vi "DMARS_Frame_v2_write.vi"(11 "DMARS":dbl[](array[numeric])) -> (0 "No DMARS string":bool, 3 "string_Out":string)   [LabVIEW 2017]
panel:
  out "SubFrame":u8
  out "milisec":u16 format="%x"
  out "sec":u16 format="%x"
  out "size(s)":i32
  out "output array":u8[](array[numeric]) format="%x"
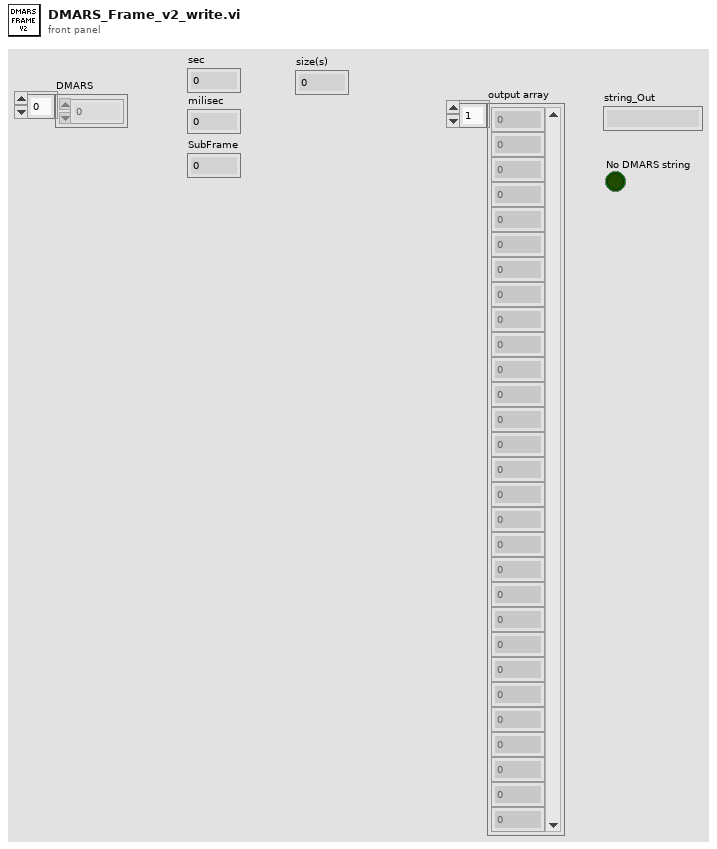
[diagram p1: front panel]
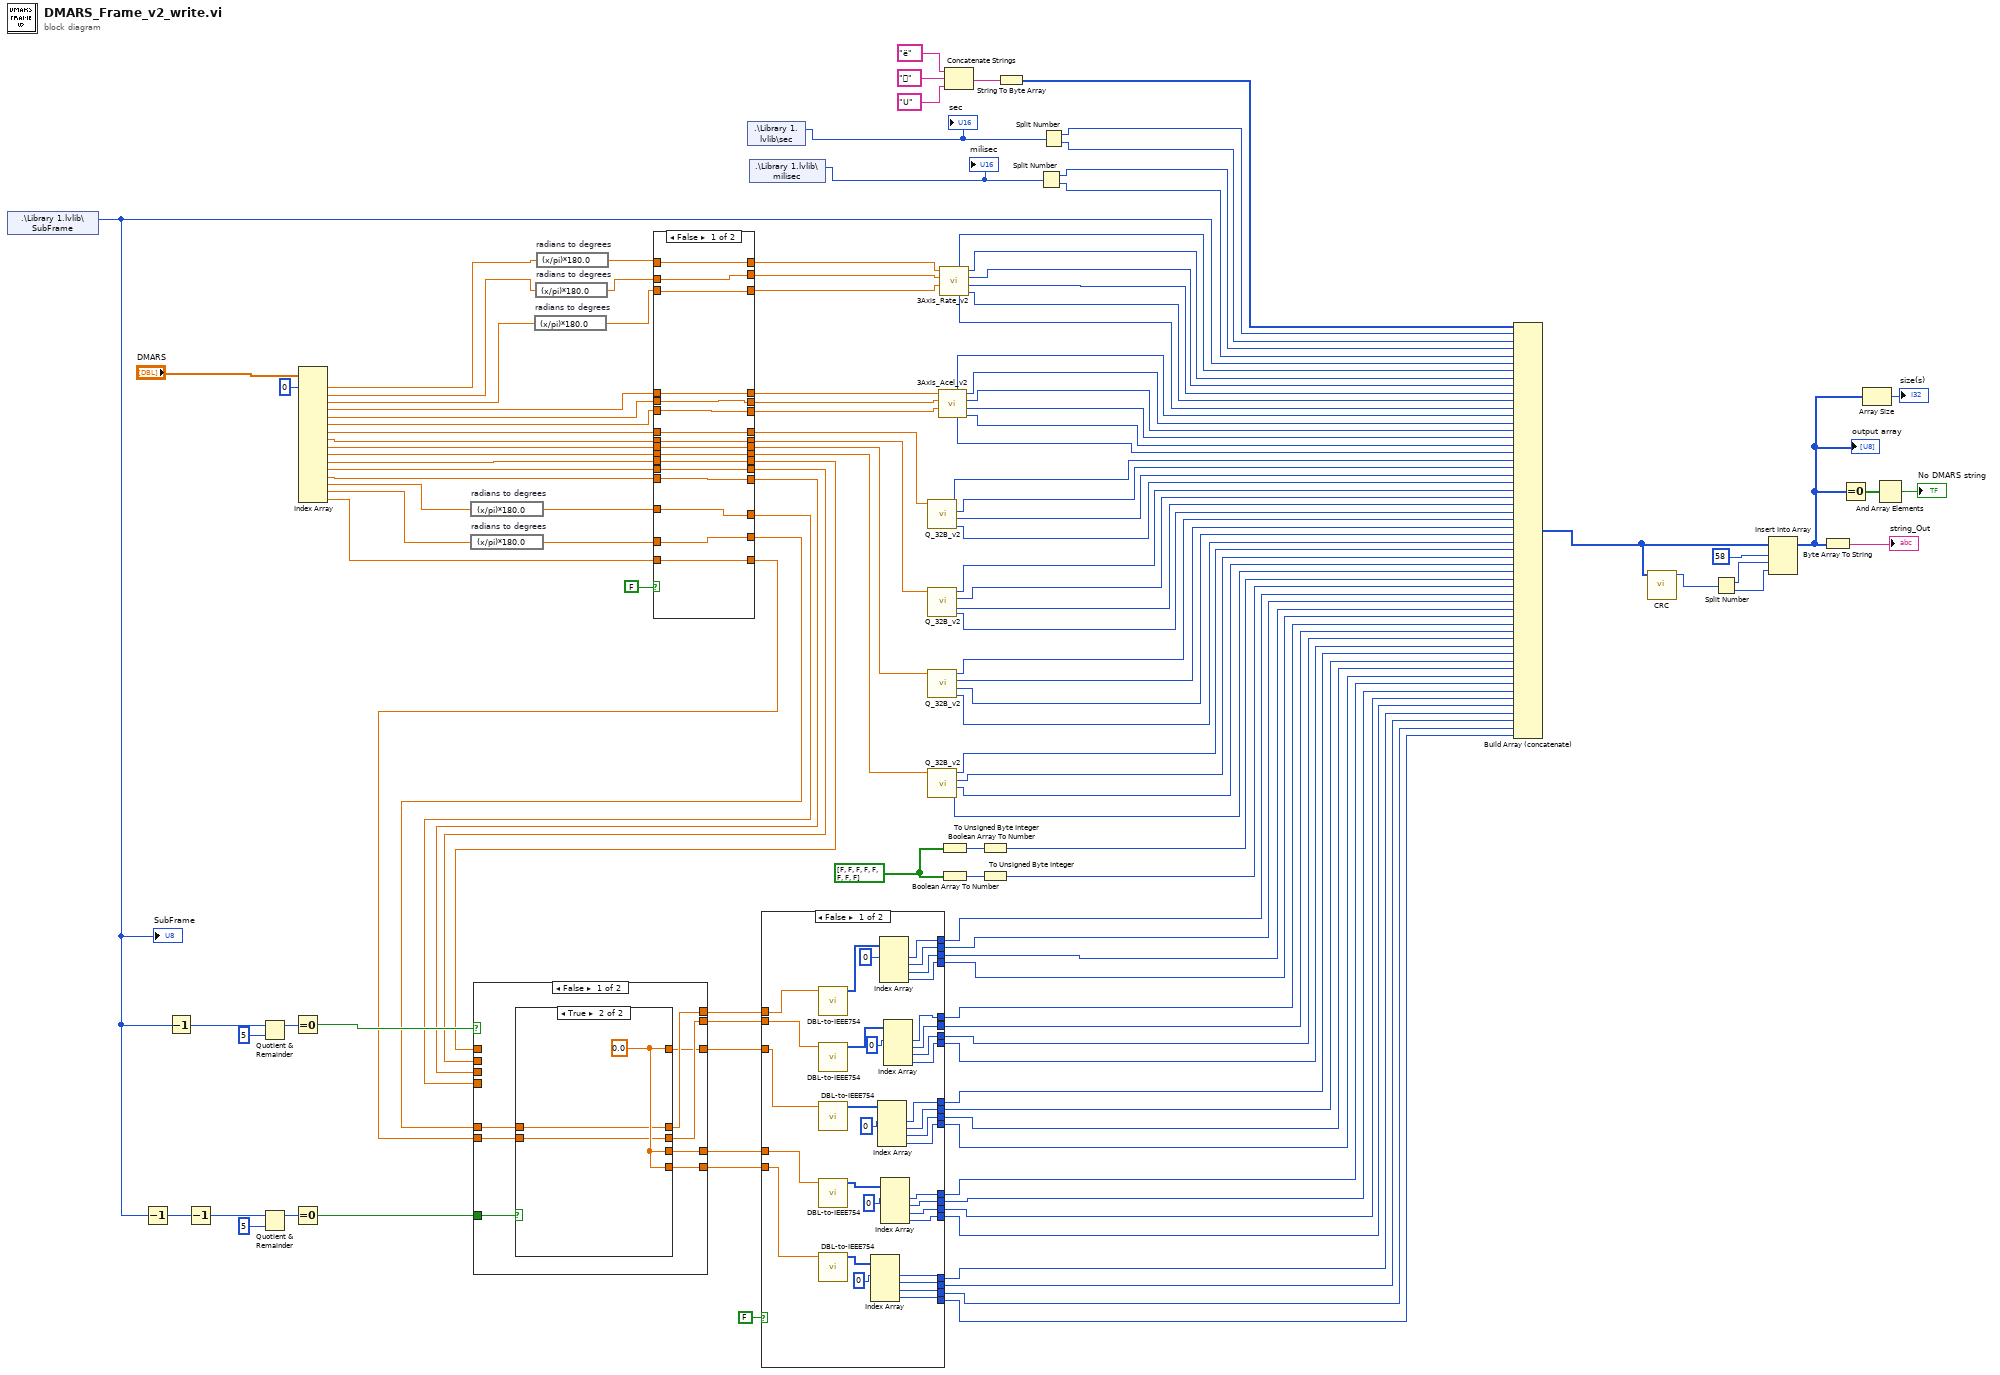
[diagram p0: block diagram]
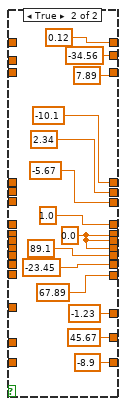
[diagram p2: hidden frame]
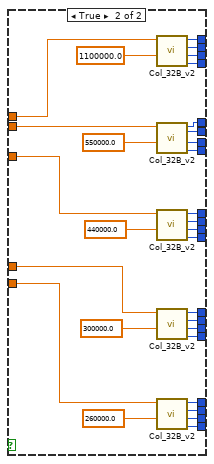
[diagram p3: hidden frame]
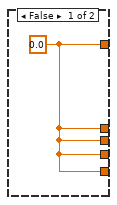
[diagram p4: hidden frame]
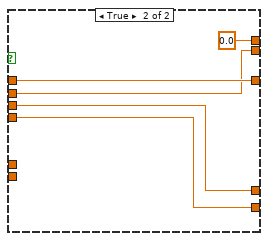
[diagram p5: hidden frame]
diagram:
  w64 = bool[] [FALSE, FALSE, FALSE, FALSE, FALSE, FALSE, FALSE, FALSE] ("Byte 36")
  n1 = shared-variable ".\\Library 1.lvlib\\SubFrame"() -> (w52:u8)  [unwired: 1 in, 1 out]
  "SubFrame" <- w52
  n2 = Decrement(x=w52) -> (x-1=w53:u8)
  n3 = Decrement(x=w52) -> (x-1=w57:u8)
  n4 = Decrement(x=w53) -> (x-1=w56:u8)
  n5 = Quotient & Remainder(x=w57, y=u8 5) -> (x-y*floor(x/y)=w59:u8)  [unwired: 1 out]
  n6 = Quotient & Remainder(x=w56, y=u8 5) -> (x-y*floor(x/y)=w55:u8)  [unwired: 1 out]
  n7 = Equal To 0?(x=w59) -> (x = 0?=w58:bool)
  n8 = Equal To 0?(x=w55) -> (x = 0?=w46:bool)
  n9 = Index Array(array="DMARS", index #1=0 ("index")) -> (element #1=w11:dbl, element #2=w9:dbl, element #3=w8:dbl, element #4=w37:dbl, element #5=w35:dbl, element #6=w33:dbl, element #7=w31:dbl, element #8=w29:dbl, element #9=w28:dbl, element #10=w25:dbl, element #11=w23:dbl, element #12=w21:dbl, element #13=w19:dbl, element #14=w45:dbl, element #15=w44:dbl, element #16=w13:dbl)  [unwired: 15 in]
  n10 = expression code="(x/pi)*180.0" "radians to degrees"(w45) -> (w17:dbl)
  n11 = expression code="(x/pi)*180.0" "radians to degrees"(w44) -> (w15:dbl)
  n12 = expression code="(x/pi)*180.0" "radians to degrees"(w8) -> (w6:dbl)
  n13 = expression code="(x/pi)*180.0" "radians to degrees"(w9) -> (w7:dbl)
  n14 = expression code="(x/pi)*180.0" "radians to degrees"(w11) -> (w10:dbl)
  n15 = case shown="False" FALSE {
    tunnel: [w146 0.12 ("Numeric")] -> w41
    tunnel: w10 -> [w146 _]
    tunnel: [w145 -34.56 ("Numeric")] -> w40
    tunnel: w7 -> [w145 _]
    tunnel: [w131 7.89 ("Numeric")] -> w39
    tunnel: w6 -> [w131 _]
    tunnel: [w144 -10.1 ("Numeric")] -> w38
    tunnel: w37 -> [w144 _]
    tunnel: [w143 2.34 ("Numeric")] -> w36
    tunnel: w35 -> [w143 _]
    tunnel: [w142 -5.67 ("Numeric")] -> w34
    tunnel: w33 -> [w142 _]
    tunnel: [w141 1.0 ("Numeric")] -> w32
    tunnel: w31 -> [w141 _]
    tunnel: [w140 w153] -> w30
    tunnel: w29 -> [w140 _]
    tunnel: w28 -> [w139 _]
    tunnel: [w139 w153] -> w27
    tunnel: [w138 w153] -> w26
    tunnel: w25 -> [w138 _]
    tunnel: [w137 89.1 ("Numeric")] -> w24
    tunnel: w23 -> [w137 _]
    tunnel: [w136 -23.45 ("Numeric")] -> w22
    tunnel: w21 -> [w136 _]
    tunnel: [w135 67.89 ("Numeric")] -> w20
    tunnel: w19 -> [w135 _]
    tunnel: [w134 -1.23 ("Numeric")] -> w18
    tunnel: w17 -> [w134 _]
    tunnel: [w133 45.67 ("Numeric")] -> w16
    tunnel: w15 -> [w133 _]
    tunnel: [w132 -8.9 ("Numeric")] -> w14
    tunnel: w13 -> [w132 _]
    frame False {
    }
    frame True {
      w153 = 0.0 ("Numeric")
    }
  }
  n16 = case shown="False" w58 {
    tunnel: w24 -> [_ w176]
    tunnel: w22 -> [_ w175]
    tunnel: w20 -> [_ w174]
    tunnel: w18 -> [_ w173]
    tunnel: [w165 0.0] -> w51
    tunnel: [w163 w176] -> w50
    tunnel: [w164 w175] -> w49
    tunnel: [w162 w174] -> w48
    tunnel: [w161 w173] -> w47
    tunnel: w46 -> [w168 _]
    tunnel: w16 -> [w167 _]
    tunnel: w14 -> [w166 _]
    frame False {
      n17 = case shown="True" w168 {
        tunnel: w167 -> [_ w171]
        tunnel: w166 -> [_ w170]
        tunnel: [w169 w171] -> w165
        tunnel: [w169 w170] -> w164
        tunnel: [w169 w172] -> w163
        tunnel: [w169 w172] -> w162
        tunnel: [w169 w172] -> w161
        frame False {
          w169 = 0.0
        }
        frame True {
          w172 = 0.0
        }
      }
    }
    frame True {
    }
  }
  n18 = shared-variable ".\\Library 1.lvlib\\sec"() -> (w63:u16)  [unwired: 1 in, 1 out]
  "sec" <- w63
  n19 = shared-variable ".\\Library 1.lvlib\\milisec"() -> (w62:u16)  [unwired: 1 in, 1 out]
  "milisec" <- w62
  n20 = case shown="False" FALSE {
    tunnel: [w181 w242] -> w125
    tunnel: [w178 w241] -> w124
    tunnel: [w179 w240] -> w123
    tunnel: [w180 w239] -> w122
    tunnel: [w182 w238] -> w121
    tunnel: [w183 w237] -> w120
    tunnel: [w184 w236] -> w119
    tunnel: [w185 w235] -> w118
    tunnel: [w190 w234] -> w117
    tunnel: [w191 w233] -> w116
    tunnel: [w192 w232] -> w115
    tunnel: [w193 w231] -> w114
    tunnel: [w196 w230] -> w113
    tunnel: [w197 w229] -> w112
    tunnel: [w198 w228] -> w111
    tunnel: [w199 w227] -> w110
    tunnel: [w203 w226] -> w109
    tunnel: [w204 w225] -> w108
    tunnel: [w205 w224] -> w107
    tunnel: [w206 w223] -> w106
    tunnel: w51 -> [w212 w222]
    tunnel: w50 -> [w210 w221]
    tunnel: w49 -> [w211 w220]
    tunnel: w48 -> [w209 w219]
    tunnel: w47 -> [w208 w218]
    frame False {
      n21 = call "DBL-to-IEEE754.vi"("Input_DBL"=w212) -> ("Output_U8"=w207:u8[])  [unwired: 10 in]
      n22 = call "DBL-to-IEEE754.vi"("Input_DBL"=w211) -> ("Output_U8"=w201:u8[])  [unwired: 10 in]
      n23 = call "DBL-to-IEEE754.vi"("Input_DBL"=w210) -> ("Output_U8"=w194:u8[])  [unwired: 10 in]
      n24 = call "DBL-to-IEEE754.vi"("Input_DBL"=w209) -> ("Output_U8"=w186:u8[])  [unwired: 10 in]
      n25 = call "DBL-to-IEEE754.vi"("Input_DBL"=w208) -> ("Output_U8"=w187:u8[])  [unwired: 10 in]
      n26 = Index Array(array=w187, index #1=0 ("index")) -> (element #1=w181:u8, element #2=w180:u8, element #3=w179:u8, element #4=w178:u8)  [unwired: 3 in]
      n27 = Index Array(array=w194, index #1=0 ("index")) -> (element #1=w193:u8, element #2=w192:u8, element #3=w191:u8, element #4=w190:u8)  [unwired: 3 in]
      n28 = Index Array(array=w207, index #1=0 ("index")) -> (element #1=w206:u8, element #2=w205:u8, element #3=w204:u8, element #4=w203:u8)  [unwired: 3 in]
      n29 = Index Array(array=w186, index #1=0 ("index")) -> (element #1=w185:u8, element #2=w184:u8, element #3=w183:u8, element #4=w182:u8)  [unwired: 3 in]
      n30 = Index Array(array=w201, index #1=0 ("index")) -> (element #1=w199:u8, element #2=w198:u8, element #3=w197:u8, element #4=w196:u8)  [unwired: 3 in]
    }
    frame True {
      n31 = call "Col_32B_v2.vi"("Ref"=1100000.0, "Col"=w222) -> ("LL"=w226:u8, "LH"=w225:u8, "HL"=w224:u8, "HH"=w223:u8)  [unwired: 6 in]
      n32 = call "Col_32B_v2.vi"("Ref"=550000.0, "Col"=w220) -> ("LL"=w230:u8, "LH"=w229:u8, "HL"=w228:u8, "HH"=w227:u8)  [unwired: 6 in]
      n33 = call "Col_32B_v2.vi"("Ref"=440000.0, "Col"=w221) -> ("LL"=w234:u8, "LH"=w233:u8, "HL"=w232:u8, "HH"=w231:u8)  [unwired: 6 in]
      n34 = call "Col_32B_v2.vi"("Ref"=300000.0, "Col"=w219) -> ("LL"=w238:u8, "LH"=w237:u8, "HL"=w236:u8, "HH"=w235:u8)  [unwired: 6 in]
      n35 = call "Col_32B_v2.vi"("Ref"=260000.0, "Col"=w218) -> ("LL"=w241:u8, "LH"=w240:u8, "HL"=w239:u8, "HH"=w242:u8)  [unwired: 6 in]
    }
  }
  n36 = call "Q_32B_v2.vi"("Q_32B"=w32) -> ("LL"=w91:u8, "HL"=w90:u8, "LH"=w89:u8, "HH"=w88:u8)  [unwired: 7 in]
  n37 = call "Q_32B_v2.vi"("Q_32B"=w30) -> ("LL"=w95:u8, "HL"=w94:u8, "LH"=w93:u8, "HH"=w92:u8)  [unwired: 7 in]
  n38 = call "Q_32B_v2.vi"("Q_32B"=w27) -> ("LL"=w99:u8, "HL"=w98:u8, "LH"=w97:u8, "HH"=w96:u8)  [unwired: 7 in]
  n39 = call "Q_32B_v2.vi"("Q_32B"=w26) -> ("LL"=w103:u8, "HL"=w102:u8, "LH"=w101:u8, "HH"=w100:u8)  [unwired: 7 in]
  n40 = call "3Axis_Acel_v2.vi"("Roll_A"=w34, "Yaw_A"=w36, "Pitch_A"=w38) -> ("RAH"=w86:u8, "YAL"=w85:u8, "YAH"=w84:u8, "PAL"=w83:u8, "RAL"=w87:u8, "PAH"=w82:u8)  [unwired: 3 in]
  n41 = call "3Axis_Rate_v2.vi"("Roll_R"=w39, "Yaw_R"=w40, "Pitch_R"=w41) -> ("RRH"=w80:u8, "YRL"=w79:u8, "YRH"=w78:u8, "PRL"=w77:u8, "RRL"=w81:u8, "PRH"=w76:u8)  [unwired: 3 in]
  n42 = Boolean Array To Number(Boolean array=w64) -> (number=w74:u32)
  n43 = Boolean Array To Number(Boolean array=w64) -> (number=w73:u32)
  n44 = Concatenate Strings("ë", "", "U") -> (w69:string)
  n45 = To Unsigned Byte Integer(number=w74) -> (unsigned 8bit integer=w104:u8)
  n46 = To Unsigned Byte Integer(number=w73) -> (unsigned 8bit integer=w105:u8)
  n47 = String To Byte Array(string=w69) -> (unsigned byte array=w75:u8[])
  n48 = Split Number(x=w62) -> (hi(x)=w127:u8, lo(x)=w128:u8)
  n49 = Split Number(x=w63) -> (hi(x)=w129:u8, lo(x)=w130:u8)
  n50 = Build Array (concatenate)(w75, w129, w130, w127, w128, w52, w76, w77, w78, w79, w80, w81, w82, w83, w84, w85, w86, w87, w88, w89, w90, w91, w92, w93, w94, w95, w96, w97, w98, w99, w100, w101, w102, w103, w104, w105, w106, w107, w108, w109, w110, w111, w112, w113, w114, w115, w116, w117, w118, w119, w120, w121, w125, w122, w123, w124) -> (w2:u8[])
  n51 = call "CRC.vi"("Array"=w2) -> ("CRC"=w1:u16)  [unwired: 10 in]
  n52 = Split Number(x=w1) -> (hi(x)=w67:u8, lo(x)=w66:u8)
  n53 = Insert Into Array(array=w2, index=58, new element #1=w67, new element #2=w66) -> (w5:u8[])
  "output array" <- w5
  n54 = Byte Array To String(unsigned byte array=w5) -> (string=→"string_Out":string)
  n55 = Equal To 0?(x=w5) -> (x = 0?=w4:bool[])
  n56 = Array Size(array=w5) -> (size(s)=→"size(s)":i32)
  n57 = And Array Elements(Boolean array=w4) -> (logical AND=→"No DMARS string":bool)
